vi "Initialize.vi"(8 "error in (no error)":errorcluster, 11 "DemoLasers in":refnum<class "DemoLasers.lvclass">) -> (0 "error out":errorcluster, 3 "DemoLasers out":refnum<class "DemoLasers.lvclass">)   [LabVIEW 2020, in "DemoLasers.lvlib" / "DemoLasers.lvclass"]
uses:
  DemoLasers.lvclass
  Hardware Abstraction Layer/Component/Laser/Laser/Laser.lvclass
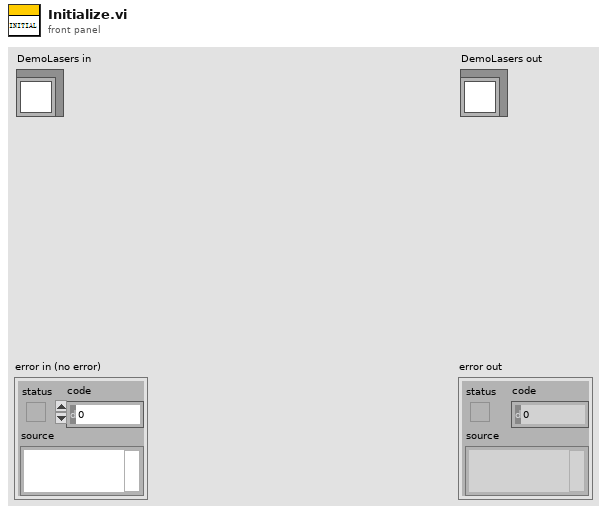
[diagram p1: front panel]
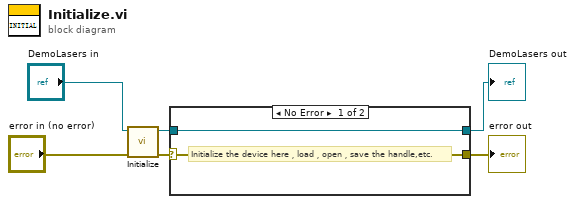
[diagram p0: block diagram]
diagram:
  n1 = call-parent "Initialize.vi"("error in (no error)"="error in (no error)", "Laser in"="DemoLasers in") -> ("error out"=w3:errorcluster, "Laser out"=w4:refnum<class "DemoLasers.lvclass">)  [unwired: 8 in]
  n2 = case shown="No Error" w3 {
    selector: w3 -> [w7 w10]
    tunnel: [w7 w10] -> w1
    tunnel: [w8 w9] -> w2
    tunnel: w4 -> [w8 w9]
    frame No Error {
      # "Initialize the device here，load，open，save the handle,etc."
    }
    frame Error {
    }
  }
  "error out" <- w1
  "DemoLasers out" <- w2
